vi "Handle Command.vi"(8 "error in (no error)":errorcluster, 9 "Data":variant, 10 "Command":string, 11 "Instrument.Lockin":refnum<class "Instrument.Lockin.lvclass">) -> (0 "error out":errorcluster, 1 "Processed Data":variant, 2 "Command":string, 3 "Instrument.Lockin out":refnum<class "Instrument.Lockin.lvclass">)   [LabVIEW 2019, in "Instrument.Lockin.lvlib" / "Instrument.Lockin.lvclass"]
uses:
  Instrument.Lockin.lvclass
  Typedefs/API/Lockin.Commands--Enum.ctl
  Typedefs/API/Lockin.Commands.Local--Enum.ctl
  <userlib>/LevyLab/Instrument Framework/Instrument Types/Lockin/Typedefs/LockinAPI.Sampling.Sampling--Cluster.ctl
  Instrument.Lockin.lvclass/Instrument.Lockin.ctl
  <userlib>/LevyLab/Instrument Framework/Instrument Types/Lockin/Typedefs/LockinAPI.Sampling.FsMode--enum.ctl
  <userlib>/LevyLab/Instrument Framework/Instrument Types/Lockin/Typedefs/LockinAPI.getState.states--enum.ctl
  <userlib>/LevyLab/Instrument Framework/Instrument Types/Lockin/Typedefs/LockinAPI.SweepData--Cluster.ctl
  Typedefs/API/Lockin.setState--cluster.ctl
  Instrument.DAQ/Typedefs/Set State-enum.ctl
  Typedefs/API/Lockin.setLogMode--cluster.ctl
  Typedefs/API/Lockin.setAO_Amp--cluster.ctl
  Typedefs/API/Lockin.setAO_DC--cluster.ctl
  Typedefs/API/Lockin.setAO_f--cluster.ctl
  Typedefs/API/Lockin.setAO_phi--cluster.ctl
  Typedefs/API/Lockin.setAO_function--cluster.ctl
  Instrument.DAQ/Typedefs/AO.Channel.Function--Enum.ctl
  Instrument.DAQ/Typedefs/AO.Channel--Cluster--Array.ctl
  Instrument.DAQ/Typedefs/AO.Channel--Cluster.ctl
  Typedefs/REF Parameter--Enum.ctl
  Typedefs/API/Lockin.setREF_f--cluster.ctl
  Typedefs/API/Lockin.setREF_phi--cluster.ctl
  Typedefs/API/Lockin.setREF_TC--cluster.ctl
  Typedefs/API/Lockin.setREF_RollOff--cluster.ctl
  Instrument.DAQ/Typedefs/REF.Channel--Cluster--Array.ctl
  Instrument.DAQ/Typedefs/REF.Channel--Cluster.ctl
  Instrument.DAQ/Typedefs/Sweep.Configuration--Cluster.ctl
  Instrument.DAQ/Typedefs/Sweep.Channel--Cluster--Array.ctl
  Instrument.DAQ/Typedefs/Sweep.Channel--Cluster.ctl
  Instrument.DAQ/Typedefs/Sweep.Pattern--Enum.ctl
  Typedefs/API/Lockin.setSweep_Time--cluster.ctl
  Typedefs/API/Lockin.setSweep_Table--cluster.ctl
  Instrument.DAQ/Typedefs/DAQ.Sampling.Sampling--Cluster.ctl
  Typedefs/API/Lockin.setSamplingFsMode--cluster.ctl
  Instrument.DAQ/Typedefs/DAQ.Sampling.Fs Mode--enum.ctl
  Instrument.DAQ/Typedefs/Channel.Gain--Cluster.ctl
  Instrument.DAQ/Typedefs/DAQ.Configuration--Cluster--Array.ctl
  Instrument.DAQ/Typedefs/DAQ.Configuration--Cluster.ctl
  Instrument.DAQ/Typedefs/DAQ.Config.AO.Range--enum.ctl
  Instrument.DAQ/Typedefs/DAQ.Config.AI.Range--enum.ctl
  Instrument.DAQ/Typedefs/DAQ.Config.AI.Coupling--enum.ctl
  Instrument.DAQ/Typedefs/PrivateEvents--DAQ.showUI.ctl
  Instrument.DAQ/Typedefs/AI.Channel--Cluster--Array.ctl
  Instrument.DAQ/Typedefs/AI.Channel--Cluster.ctl
  Instrument.DAQ/Typedefs/Simulation Mode--enum.ctl
  Typedefs/Offset Mode--Enum.ctl
  Instrument.DAQ/Typedefs/PrivateEvents--DAQ.setCalibration.ctl
  Instrument.DAQ/Typedefs/Configuration.Prefilter--Cluster.ctl
  Instrument.DAQ/Typedefs/Configuration.LinkFrequencies--Cluster.ctl
  Instrument.DAQ/Typedefs/Configuration.AmplitudeLimit--Cluster.ctl
  Typedefs/API/Lockin.setSamplingMode--cluster.ctl
  Instrument.DAQ/Typedefs/DAQ.Sampling.Sample Mode--Ring.ctl
  afc408c1-4a47-494c-817e-7b9f9bb33729.vi
  a7ccf487-04bf-437f-bc58-012293c091eb.vi
  06f5bff1-b823-416c-a758-fc672ecfcc99.vi
  029a7bc4-99e9-4f65-b437-c26585c9cd40.vi
  95117756-58c8-4cf5-b4a1-eea4f9571e2f.vi
  d527b0ad-2cbe-40d7-81d2-49d8d0078832.vi
  c6561379-f98d-4793-93aa-fc4f7b6fa2da.vi
  f7b28b50-f868-4d06-8d90-790d331e6843.vi
  3b890341-4124-4342-9d75-403cba162ea7.vi
  efd52b93-d691-4a9b-b54f-f4c6778ec2a4.vi
  1b48001d-6f4c-40ce-9883-2cfdfc5b0066.vi
  2465c698-e437-4a4f-8860-a626a4e5f6de.vi
  451a16e7-7f0f-4872-98b2-f896a68061ac.vi
  ce862ac6-3818-4682-989c-38fcf43d7c0a.vi
  0f1e83ab-c55c-46b9-bca3-9d617c6a026d.vi
  c46d61d8-ad78-4a4f-bd83-bba7d42c3393.vi
  06811b67-d74b-4972-af3b-9250fa170671.vi
  148daf87-aacf-4ea0-9f45-6b19ec731a12.vi
  b666889e-e9d3-40fa-bff7-b740bef29075.vi
  7fa0c9c7-d96f-42eb-b083-8fec20da1e25.vi
  2eef0b96-7480-46b2-a416-598848f5f946.vi
  4baefe16-dd55-4900-a34f-f85402a43af0.vi
  bf5afc16-6b2f-47bd-9035-54b404507785.vi
  df248ea2-cdbc-4a64-a66c-167358fcc18f.vi
  f4b2f717-a3e3-4701-aa1a-36f1ad587562.vi
  cb03029c-6dea-422e-9ff0-c01ba24202a7.vi
  ea7ae40a-427f-4df9-8330-54c2df2a5be0.vi
  d5077292-e533-4b52-a4d7-ebb5f6280e78.vi
  be7fa38f-04e0-4644-9c08-a6c1d8484273.vi
  228c5f99-5a8a-4ac9-8c3f-6c80f04cbb43.vi
  d91f965c-decf-4ad0-9779-3bd2f4599088.vi
  d9adaec0-ad08-4a9e-8669-6c491ae292cb.vi
  acd43294-18b9-4ae6-b527-f08772f90be2.vi
  6a1e6d83-5b10-4acb-978a-0f1ae3d31a35.vi
  847e6f07-fde4-45b3-9907-c341240c9864.vi
  b8b9aa39-8fbe-4465-abb6-4b3c602a596b.vi
  <vilib>/JDP Science/JSONtext/JSON text to Variant.vi
  <vilib>/JDP Science/JSONtext/LVClass Serializer/JSONtext LVClass Serializer.lvclass
  <userlib>/LevyLab/Instrument Framework/Instrument Types/Lockin/Instrument.LockinAPI.lvclass
  Instrument.DAQ/Instrument.DAQ.lvclass
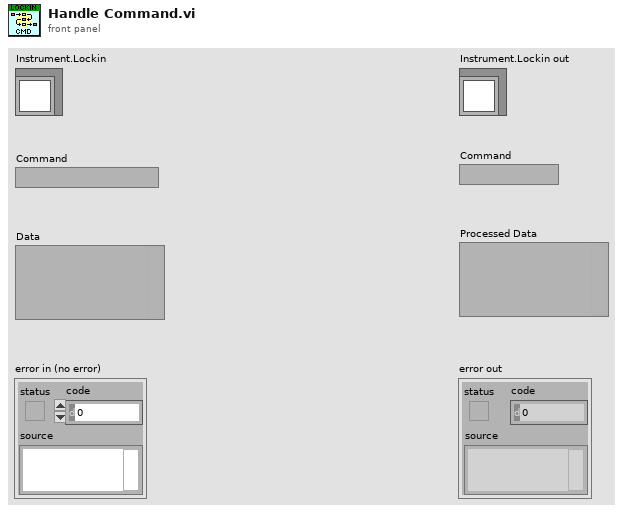
[diagram p1: front panel]
types:
  T1 = typedef "Instrument.Lockin.lvlib/Instrument.Lockin.lvclass/Lockin.Commands.Local--Enum.ctl" = enum16{"autoConfigureDAQ", "setSimulationMode", "zeroPhase", "setCalibration", "setPreFilter", "setLinkFrequencies", "setLimitAmplitude", "setLimitDC", "setSamplingDecimationPreDSP", "setSamplingDecimationPostDSP", "setSamplingMode", "setSamplingFsMultiplier", "setSamplingFsOutput", "setSamplingRefreshRate", "setData_State", "setData_DAQ", "setData_Sampling", "setData_Waveforms", "setData_Results", "setData_SweepWaveforms", "setData_AIChannels", "setData_AOChannels", "setData_REFChannels", "setData_InputGain", "setData_OutputGain", "showUI", "setAI", "setOffset", "setOffsetMode"}
  T2 = typedef "Instrument.Lockin.lvlib/Instrument.Lockin.lvclass/Lockin.Commands--Enum.ctl" = enum16{"setAO", "setAO_Amplitude", "setAO_DC", "setAO_Frequency", "setAO_Phase", "setAO_Function", "setREF", "setREF_Frequency", "setREF_Phase", "setREF_TC", "setREF_Roll-Off", "setDAQ", "setSampling", "setState", "getState", "getAO", "getAI", "getResults", "getSampling", "getAOconfig", "getREFconfig", "setInputGain", "setOutputGain", "getInputGain", "getOutputGain", "setSamplingFsMode", "getSamplingFsMode", "setSweep", "setSweep_Time", "setSweep_Table", "getStatus", "getSweepResults", "getSweepWaveforms", "startLogging", "stopLogging"}
  T3 = typedef "Instrument.LockinAPI.lvclass/LockinAPI.Sampling.Sampling--Cluster.ctl" = cluster{"Fs":dbl, "#s":i32}
  T4 = typedef "Instrument.LockinAPI.lvclass/LockinAPI.getState.states--enum.ctl" = enum16{"idle", "created", "started", "stopped", "sweeping"}
  T5 = typedef "Instrument.LockinAPI.lvclass/LockinAPI.SweepData--Cluster.ctl" = cluster{"AO":waveform(dbl)[], "AI":waveform(dbl)[], "X":waveform(dbl)[], "Y":waveform(dbl)[]}
  T6 = typedef "Instrument.Lockin.lvlib/Instrument.Lockin.lvclass/Lockin.setState--cluster.ctl" = cluster{"State":T7}
  T7 = typedef "Instrument.Lockin.lvlib/Instrument.DAQ.lvclass/Set State-enum.ctl" = enum16{"start", "stop", "reset", "start sweep", "stop sweep"}
  T8 = typedef "Instrument.Lockin.lvlib/Instrument.Lockin.lvclass/Lockin.setLogMode--cluster.ctl" = cluster{"interval":u32}
  T9 = enum16{"Amplitude", "DC", "Frequency", "Phase", "Function"}
  T10 = typedef "Instrument.Lockin.lvlib/Instrument.Lockin.lvclass/Lockin.setAO_Amp--cluster.ctl" = cluster{"Channel":i32, "Amplitude":dbl}
  T11 = typedef "Instrument.Lockin.lvlib/Instrument.Lockin.lvclass/Lockin.setAO_DC--cluster.ctl" = cluster{"Channel":i32, "DC":dbl}
  T12 = typedef "Instrument.Lockin.lvlib/Instrument.Lockin.lvclass/Lockin.setAO_f--cluster.ctl" = cluster{"Channel":i32, "Frequency":dbl}
  T13 = typedef "Instrument.Lockin.lvlib/Instrument.Lockin.lvclass/Lockin.setAO_phi--cluster.ctl" = cluster{"Channel":i32, "Phase":dbl}
  T14 = typedef "Instrument.Lockin.lvlib/Instrument.Lockin.lvclass/Lockin.setAO_function--cluster.ctl" = cluster{"Channel":i32, "Function":T15}
  T15 = typedef "Instrument.Lockin.lvlib/Instrument.DAQ.lvclass/AO.Channel.Function--Enum.ctl" = enum16{"Sine", "Triangle", "Square"}
  T16 = typedef "Instrument.Lockin.lvlib/Instrument.DAQ.lvclass/AO.Channel--Cluster--Array.ctl" = T17[]
  T17 = typedef "Instrument.Lockin.lvlib/Instrument.DAQ.lvclass/AO.Channel--Cluster.ctl" = cluster{"Enable?":bool, "Channel":i32, "Amplitude":dbl, "Offset":dbl, "Frequency":dbl, "Phase":dbl, "Function":T15, "Sweeping?":bool}
  T18 = typedef "Instrument.Lockin.lvlib/Instrument.Lockin.lvclass/Lockin.setREF_f--cluster.ctl" = cluster{"Channel":i32, "Frequency":dbl}
  T19 = typedef "Instrument.Lockin.lvlib/Instrument.Lockin.lvclass/REF Parameter--Enum.ctl" = enum16{"Frequency", "Phase", "Time Constant", "RollOff"}
  T20 = typedef "Instrument.Lockin.lvlib/Instrument.Lockin.lvclass/Lockin.setREF_phi--cluster.ctl" = cluster{"Channel":i32, "Phase":dbl}
  T21 = typedef "Instrument.Lockin.lvlib/Instrument.Lockin.lvclass/Lockin.setREF_TC--cluster.ctl" = cluster{"Channel":i32, "TC":dbl}
  T22 = typedef "Instrument.Lockin.lvlib/Instrument.Lockin.lvclass/Lockin.setREF_RollOff--cluster.ctl" = cluster{"Channel":i32, "Roll-Off":i32}
  T23 = typedef "Instrument.Lockin.lvlib/Instrument.DAQ.lvclass/REF.Channel--Cluster--Array.ctl" = T24[]
  T24 = typedef "Instrument.Lockin.lvlib/Instrument.DAQ.lvclass/REF.Channel--Cluster.ctl" = cluster{"Enable?":bool, "Channel":i32, "Frequency":dbl, "Phase":dbl, "TC":dbl, "Roll-Off":i32}
  T25 = typedef "Instrument.Lockin.lvlib/Instrument.Lockin.lvclass/Lockin.setSweep_Time--cluster.ctl" = cluster{"SweepTime":dbl}
  T26 = typedef "Instrument.Lockin.lvlib/Instrument.Lockin.lvclass/Lockin.setSweep_Table--cluster.ctl" = cluster{"Channel":i32, "Table":dbl[]}
  T27 = typedef "Instrument.Lockin.lvlib/Instrument.DAQ.lvclass/DAQ.Sampling.Sampling--Cluster.ctl" = cluster{"Fs":dbl, "#s":i32}
  T28 = typedef "Instrument.Lockin.lvlib/Instrument.Lockin.lvclass/Lockin.setSamplingFsMode--cluster.ctl" = cluster{"FsMode":T29}
  T29 = typedef "Instrument.Lockin.lvlib/Instrument.DAQ.lvclass/DAQ.Sampling.Fs Mode--enum.ctl" = enum16{"Manual", "Auto Fs", "Max Fs"}
  T30 = typedef "Instrument.Lockin.lvlib/Instrument.DAQ.lvclass/Channel.Gain--Cluster.ctl" = cluster{"Channel":string, "Gain":dbl}
  T31 = typedef "Instrument.Lockin.lvlib/Instrument.DAQ.lvclass/DAQ.Configuration--Cluster--Array.ctl" = T32[]
  T32 = typedef "Instrument.Lockin.lvlib/Instrument.DAQ.lvclass/DAQ.Configuration--Cluster.ctl" = cluster{"Device":string, "AO.Ch":string, "AO.Range":T33, "AI.Ch":string, "AI.Range":T34, "AI.Coupling":T35}
  T33 = typedef "Instrument.Lockin.lvlib/Instrument.DAQ.lvclass/DAQ.Config.AO.Range--enum.ctl" = enum16{"±0.1", "±1.0", "±10.0"}
  T34 = typedef "Instrument.Lockin.lvlib/Instrument.DAQ.lvclass/DAQ.Config.AI.Range--enum.ctl" = enum16{"±0.316", "±1.00", "±3.16", "±10.0", "±31.6", "±42.4"}
  T35 = typedef "Instrument.Lockin.lvlib/Instrument.DAQ.lvclass/DAQ.Config.AI.Coupling--enum.ctl" = u16
  T36 = typedef "Instrument.Lockin.lvlib/Instrument.DAQ.lvclass/PrivateEvents--DAQ.showUI.ctl" = bool
  T37 = typedef "Instrument.Lockin.lvlib/Instrument.DAQ.lvclass/AI.Channel--Cluster--Array.ctl" = T38[]
  T38 = typedef "Instrument.Lockin.lvlib/Instrument.DAQ.lvclass/AI.Channel--Cluster.ctl" = cluster{"Enable?":bool, "Channel":i32, "References":i32[]}
  T39 = typedef "Instrument.Lockin.lvlib/Instrument.DAQ.lvclass/Simulation Mode--enum.ctl" = enum16{"AI = HW simulated", "AI = noise*AO", "AI = waveguide"}
  T40 = typedef "Instrument.Lockin.lvlib/Instrument.Lockin.lvclass/Offset Mode--Enum.ctl" = enum16{"Measure", "Remove"}
  T41 = typedef "Instrument.Lockin.lvlib/Instrument.DAQ.lvclass/PrivateEvents--DAQ.setCalibration.ctl" = enum16{"Check", "Calibrate"}
  T42 = typedef "Instrument.Lockin.lvlib/Instrument.DAQ.lvclass/Configuration.Prefilter--Cluster.ctl" = cluster{"60 Hz":bool, "Low Pass":bool, "Low Pass Cutoff (Hz)":dbl}
  T43 = typedef "Instrument.Lockin.lvlib/Instrument.DAQ.lvclass/Configuration.LinkFrequencies--Cluster.ctl" = cluster{"Link?":bool, "Frequency (Hz)":dbl}
  T44 = typedef "Instrument.Lockin.lvlib/Instrument.Lockin.lvclass/Lockin.setSamplingMode--cluster.ctl" = cluster{"SampleMode":T45}
  T45 = typedef "Instrument.Lockin.lvlib/Instrument.DAQ.lvclass/DAQ.Sampling.Sample Mode--Ring.ctl" = i32
  T46 = typedef "Instrument.LockinAPI.lvclass/LockinAPI.Sampling.FsMode--enum.ctl" = enum16{"Manual", "Auto Fs", "Max Fs"}
  T47 = typedef "Instrument.Lockin.lvlib/Instrument.DAQ.lvclass/Get State-enum.ctl" = enum16{"idle", "created", "started", "stopped", "sweeping"}
  T48 = typedef "Instrument.Lockin.lvlib/Instrument.DAQ.lvclass/Channel.Gain--Cluster--Array.ctl" = T30[]
  T49 = typedef "Instrument.Lockin.lvlib/Instrument.DAQ.lvclass/Results--Cluster.ctl" = cluster{"Time Stamp":timestamp, "Results (Dictionary)":cluster{"key":string, "value":dbl}[]}
  T50 = typedef "Instrument.Lockin.lvlib/Instrument.DAQ.lvclass/Sweep.Configuration--Cluster.ctl" = cluster{"Sweep Time (s)":dbl, "Initial Wait (s)":dbl, "Return to Start":bool, "Channels":T51}
  T51 = typedef "Instrument.Lockin.lvlib/Instrument.DAQ.lvclass/Sweep.Channel--Cluster--Array.ctl" = T52[]
  T52 = typedef "Instrument.Lockin.lvlib/Instrument.DAQ.lvclass/Sweep.Channel--Cluster.ctl" = cluster{"Enable?":bool, "Channel":u16, "Start":dbl, "End":dbl, "Pattern":T53, "Table":dbl[]}
  T53 = typedef "Instrument.Lockin.lvlib/Instrument.DAQ.lvclass/Sweep.Pattern--Enum.ctl" = enum16{"Ramp /", "Ramp /\\", "Smooth Ramp _/", "Smooth Ramp _/\\_", "Table"}
  T54 = typedef "Instrument.Lockin.lvlib/Instrument.DAQ.lvclass/DAQ.Sampling--Cluster.ctl" = cluster{"Sampling":T27, "sample mode":i32, "Fs Mode":T29, "Fs Multiplier":dbl, "Refresh Rate (Hz)":dbl, "Decimation.PreDSP":i32, "Decimation.PostDSP":i32, "Fs.Output":dbl}
  T55 = typedef "Instrument.Lockin.lvlib/Instrument.DAQ.lvclass/DAQ.Config.AO--Cluster--Array.ctl" = T56[]
  T56 = typedef "Instrument.Lockin.lvlib/Instrument.DAQ.lvclass/DAQ.Config.AO--Cluster.ctl" = cluster{"Channels":tag, "Range":T33, "output terminal configuration":i32, "Type":T57}
  T57 = typedef "Instrument.Lockin.lvlib/Instrument.DAQ.lvclass/DAQ.Type--enum.ctl" = enum16{"None", "USB-4431", "PXI-446x"}
  T58 = typedef "Instrument.Lockin.lvlib/Instrument.DAQ.lvclass/DAQ.Config.AI--Cluster--Array.ctl" = T59[]
  T59 = typedef "Instrument.Lockin.lvlib/Instrument.DAQ.lvclass/DAQ.Config.AI--Cluster.ctl" = cluster{"Channels":tag, "Coupling":T35, "Range":T34, "input terminal configuration":i32, "Type":T57}
  T60 = typedef "Instrument.Lockin.lvlib/Instrument.DAQ.lvclass/PublicEvents--DAQ.getWaveforms.ctl" = cluster{"AO_wfm":waveform(dbl)[], "AI_wfm":waveform(dbl)[], "Ref_X_wfm":waveform(dbl)[], "Ref_Y_wfm":waveform(dbl)[], "X_wfm":waveform(dbl)[], "Y_wfm":waveform(dbl)[]}
  T61 = typedef "Instrument.Lockin.lvlib/Instrument.DAQ.lvclass/PublicEvents--DAQ.getSweepWaveforms.ctl" = cluster{"AO_wfm":waveform(dbl)[], "AI_wfm":waveform(dbl)[], "X_wfm":waveform(dbl)[], "Y_wfm":waveform(dbl)[]}
  T62 = typedef "Instrument.Lockin.lvlib/Instrument.DAQ.lvclass/Configuration.AmplitudeLimit--Cluster.ctl" = cluster{"Limit?":bool, "Limit (V)":dbl}
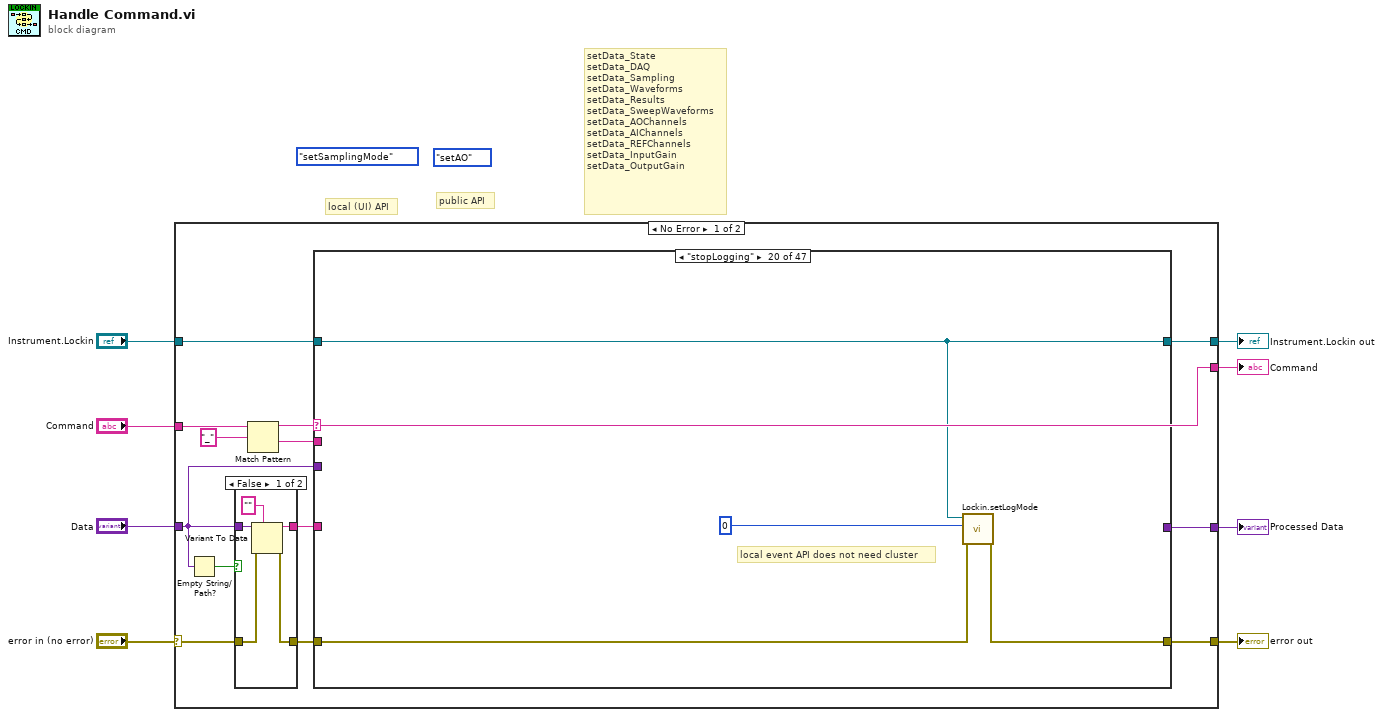
[diagram p0: block diagram]
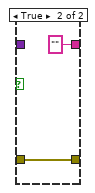
[diagram p2: hidden frame]
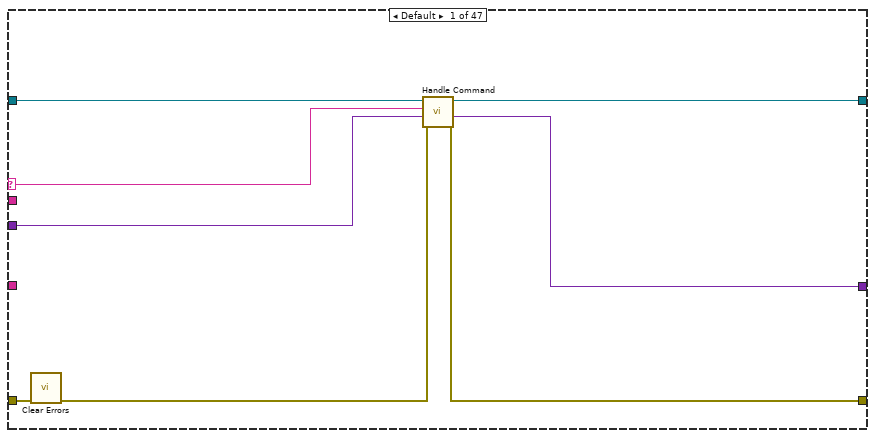
[diagram p3: hidden frame]
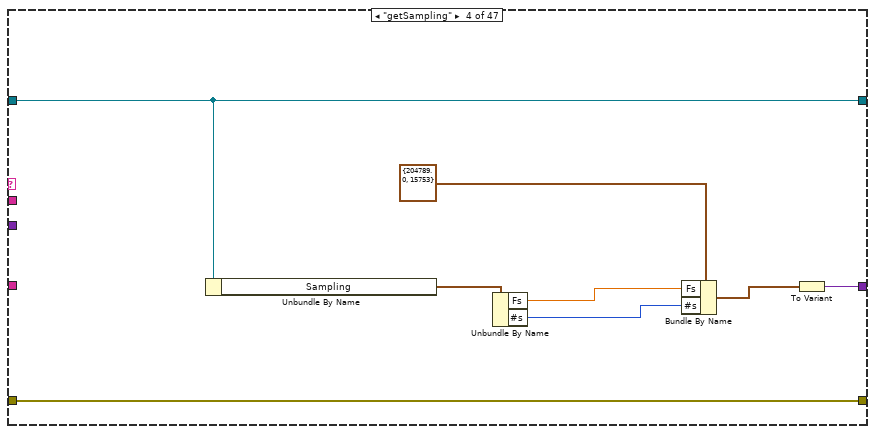
[diagram p6: hidden frame]
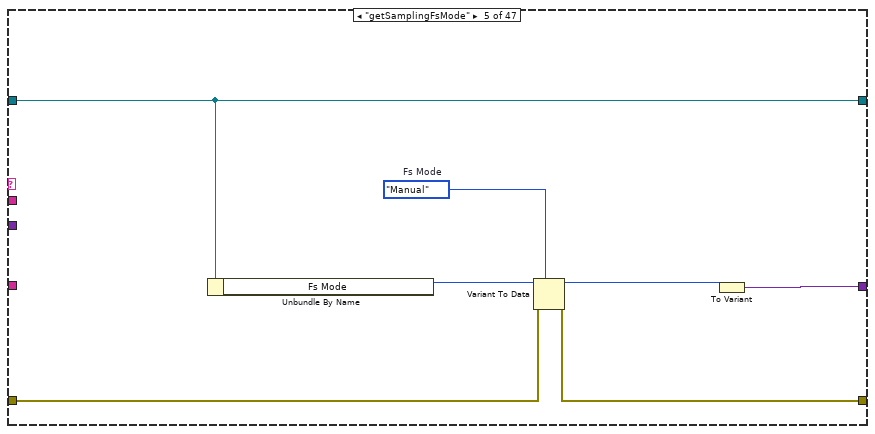
[diagram p7: hidden frame]
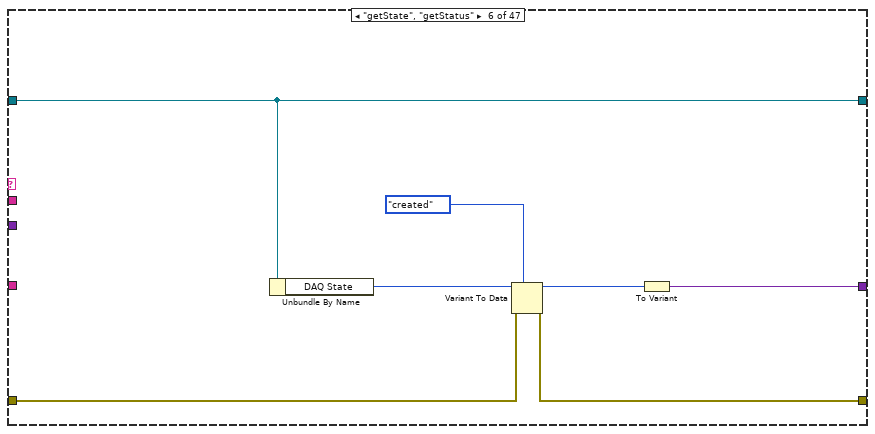
[diagram p8: hidden frame]
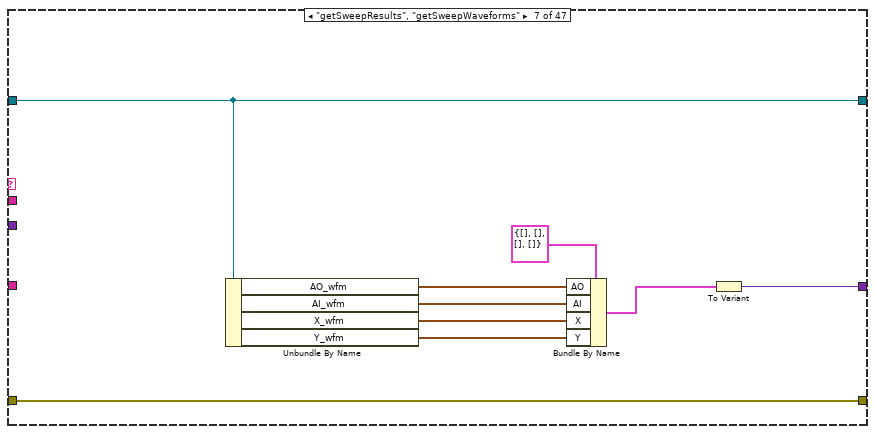
[diagram p9: hidden frame]
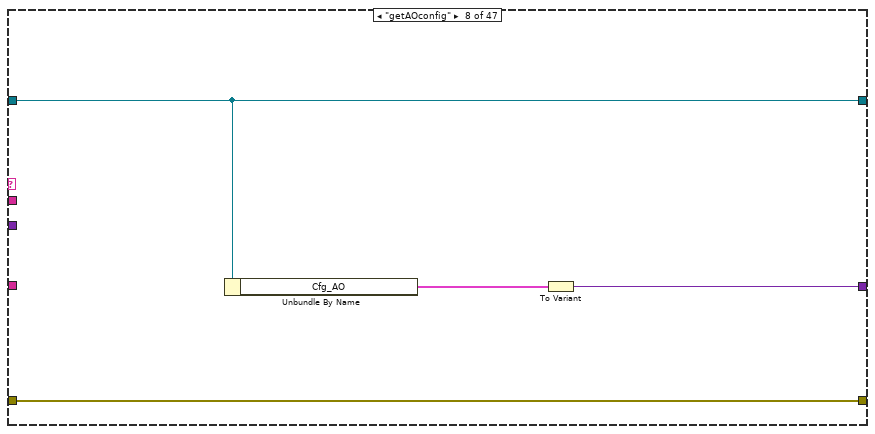
[diagram p10: hidden frame]
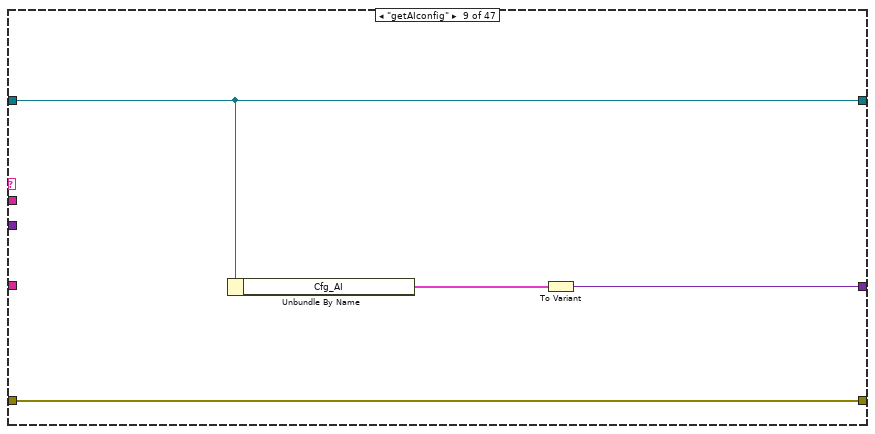
[diagram p11: hidden frame]
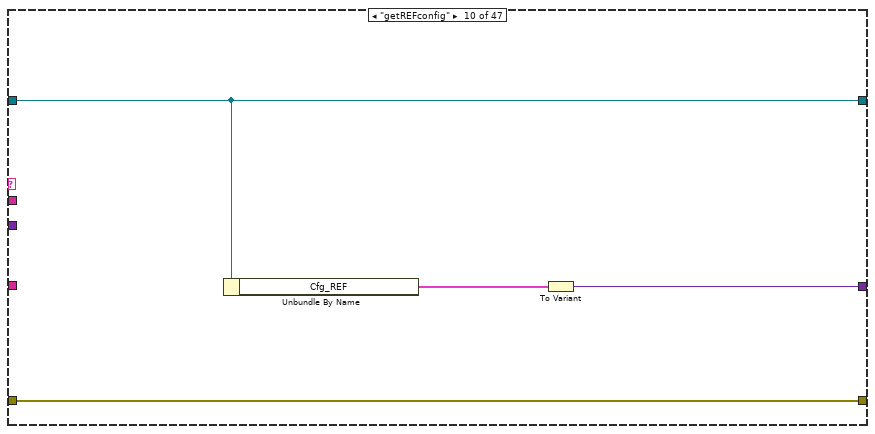
[diagram p12: hidden frame]
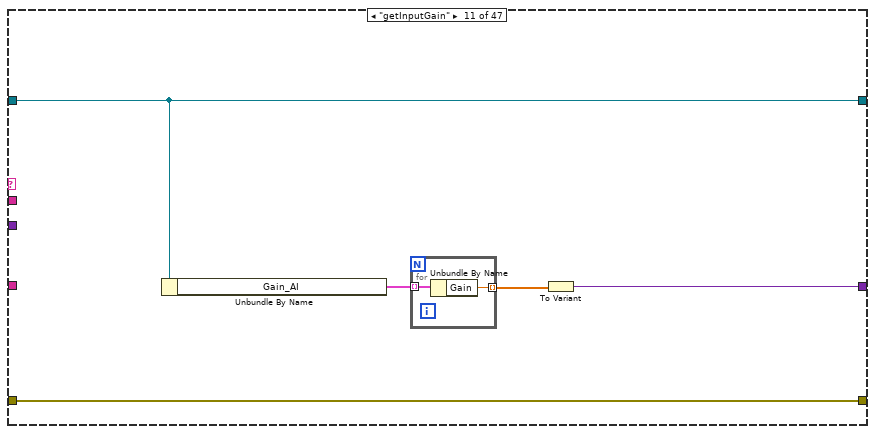
[diagram p13: hidden frame]
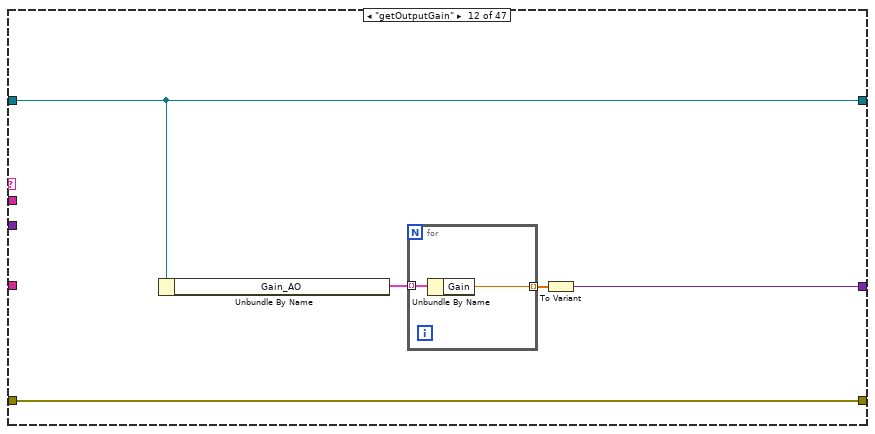
[diagram p14: hidden frame]
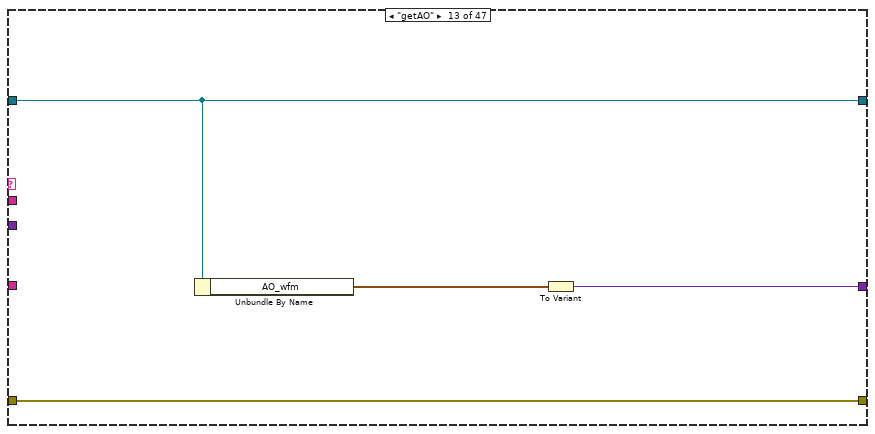
[diagram p15: hidden frame]
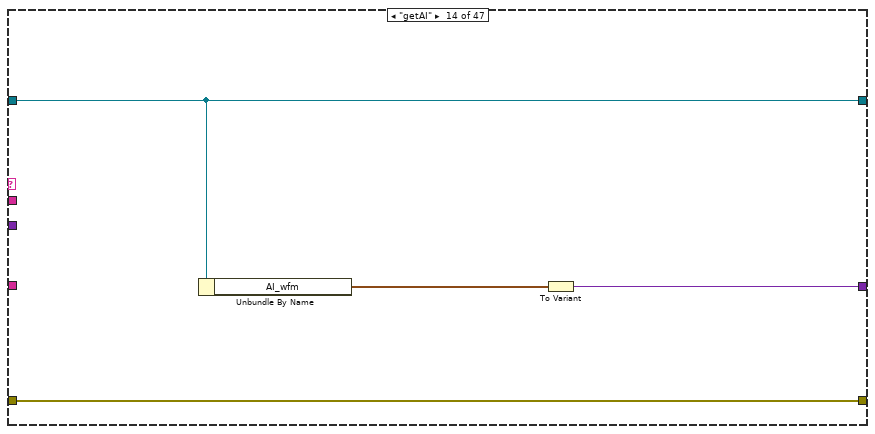
[diagram p16: hidden frame]
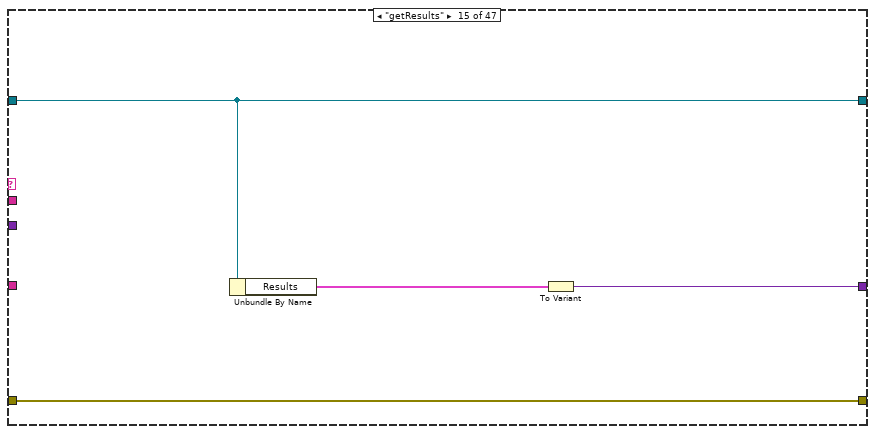
[diagram p17: hidden frame]
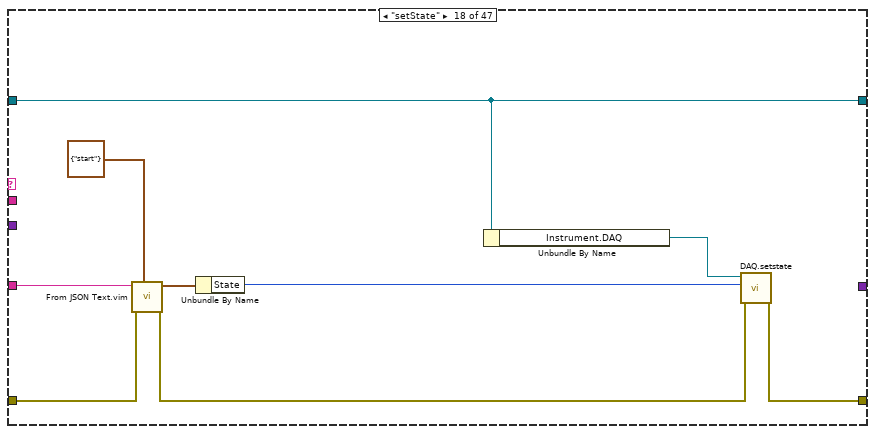
[diagram p20: hidden frame]
diagram:
  (unwired) Lockin.Commands.Local--Enum."setSamplingMode" ("Enum")
  (unwired) Lockin.Commands--Enum."setAO" ("Enum")
  # "setData_State\nsetData_DAQ\nsetData_Sampling\nsetData_Waveforms\nsetData_Results\nsetData_SweepWaveforms\nsetData_AOChannels\nsetData_AIChannels\nsetData_REFChannels\nsetData_InputGain\nsetData_OutputGain"
  # "local (UI) API"
  # "public API"
  n1 = case shown="No Error" "error in (no error)" {
    selector: "error in (no error)" -> [w17 w662]
    tunnel: [w18 w662] -> w7
    tunnel: [w20 w661] -> w6
    tunnel: "Instrument.Lockin" -> [w21 w661]
    tunnel: "Command" -> [w12 w660]
    tunnel: [w19 variant] -> w5
    tunnel: "Data" -> [w9 _]
    tunnel: [w11 w660] -> w3
    frame No Error {
      n2 = Empty String/Path?(string/path=w9) -> (empty?=w10:bool)
      n3 = case shown="False" w10 {
        tunnel: w17 -> [w26 w27]
        tunnel: [w24 ""] -> w16
        tunnel: [w23 w27] -> w13
        tunnel: w9 -> [w22 _]
        frame False {
          n4 = Variant To Data(error in=w26, type="", Variant=w22) -> (data=w24:string, error out=w23:errorcluster)
        }
        frame True {
        }
      }
      n5 = Match Pattern(string=w12, regular expression="_") -> (before substring=w11:string, after substring=w14:string)  [unwired: 1 in, 2 out]
      n6 = case shown="\"stopLogging\"" w11 {
        selector: w11 -> [w31 _ _ _ _ _ _ _ _ _ _ _ _ _ _ _ _ _ _ _ _ _ _ _ _ _ _ _ _ _ _ _ _ _ _ _ _ _ _ _ _ _ _ _ _ _ _]
        tunnel: w21 -> [w36 w38 w40 w46 w54 w61 w69 w72 w76 w80 w86 w93 w98 w102 w106 w111 w113 w117 w126 w134 w139 w213 w272 w304 w319 w328 w346 w365 w382 w395 w397 w411 w419 w526 w539 w549 w558 w567 w574 w586 w596 w604 w614 w628 w638 w648 w658]
        tunnel: [w34 w38 w40 w46 w54 w61 w69 w72 w76 w80 w86 w93 w98 w102 w106 w111 w113 w117 w126 w134 w137 w208 w276 w303 w316 w329 w347 w366 w381 w395 w397 w405 w415 w526 w538 w549 w558 w567 w575 w587 w597 w603 w613 w625 w635 w645 w655] -> w20
        tunnel: [w35 _ _ w48 w55 w62 w71 w74 w78 w82 w88 w95 w101 w105 w109 _ _ _ _ _ _ _ _ _ _ _ _ _ _ _ _ _ _ _ _ w540 _ _ _ _ _ _ _ _ _ _ _] -> w19
        tunnel: w16 -> [_ _ _ _ _ _ _ _ _ _ _ _ _ _ _ _ _ w122 w130 _ w143 w216 w280 w310 w321 w334 w352 w370 w393 _ w403 w413 w417 _ w533 w546 _ w564 w571 w582 w592 w602 w612 w623 w632 w642 w653]
        tunnel: [w32 w37 w39 w47 w50 w57 w70 w73 w77 w81 w87 w94 w100 w104 w108 w110 w112 w118 w123 w133 w140 w209 w277 w306 w314 w330 w348 w367 w387 w394 w398 w407 w414 w528 w534 w547 w556 w565 w576 w583 w593 w605 w615 w624 w634 w644 w654] -> w18
        tunnel: w14 -> [_ _ _ _ _ _ _ _ _ _ _ _ _ _ _ _ _ _ _ _ w138 w214 w273 _ _ _ _ _ _ _ _ _ w418 _ _ _ _ _ _ _ _ _ _ _ _ _ _]
        tunnel: w13 -> [w33 w37 w39 w47 w49 w56 w70 w73 w77 w81 w87 w94 w100 w104 w108 w110 w112 w121 w129 w131 w142 w215 w279 w308 w320 w333 w351 w369 w392 w394 w400 w412 w416 w527 w532 w543 w557 w560 w569 w580 w589 w601 w611 w622 w630 w641 w650]
        tunnel: w9 -> [w30 _ _ _ _ _ _ _ _ _ _ _ _ _ _ _ _ _ _ _ _ _ _ _ _ _ _ _ _ _ _ _ _ _ _ _ _ _ _ _ _ _ _ _ _ _ _]
        frame Default {
          n7 = call <vilib>:"Clear Errors.vi"("error in (no error)"=w33) -> ("error out"=w29:errorcluster)  [unwired: 5 in, 1 out]
          n8 = call-parent "Handle Command.vi"("error in (no error)"=w29, "params in"=w30, "command"=w31, "Instrument in"=w36) -> ("error out"=w32:errorcluster, "processed data"=w35:variant, "Instrument out"=w34:refnum<class "Instrument.Lockin.lvclass">)  [unwired: 4 in, 1 out]
        }
        frame "----------PUBLIC API----------" {
        }
        frame "----------GET METHODS----------" {
        }
        frame "getSampling" {
          n9 = Unbundle By Name(w46) -> ("Sampling"=w44:T27)
          n10 = Unbundle By Name(w44) -> ("Fs"=w43:dbl, "#s"=w42:i32)
          n11 = Bundle By Name(cluster=T3 {"Fs"=204789.0, "#s"=15753} ("sampling"), "Fs"=w43, "#s"=w42) -> (w41:T3)
          n12 = To Variant(anything=w41) -> (Variant=w48:variant)
        }
        frame "getSamplingFsMode" {
          w52 = LockinAPI.Sampling.FsMode--enum."Manual"  # Fs Mode
          n13 = Unbundle By Name(w54) -> ("Fs Mode"=w53:T29)
          n14 = Variant To Data(error in=w49, type=w52, Variant=w53) -> (data=w51:T46, error out=w50:errorcluster)
          n15 = To Variant(anything=w51) -> (Variant=w55:variant)
        }
        frame "getState", "getStatus" {
          n16 = Unbundle By Name(w61) -> ("DAQ State"=w59:T47)
          n17 = Variant To Data(error in=w56, type=LockinAPI.getState.states--enum."created" ("getState.states"), Variant=w59) -> (data=w58:T4, error out=w57:errorcluster)
          n18 = To Variant(anything=w58) -> (Variant=w62:variant)
        }
        frame "getSweepResults", "getSweepWaveforms" {
          n19 = Unbundle By Name(w69) -> ("AO_wfm"=w67:waveform(dbl)[], "AI_wfm"=w66:waveform(dbl)[], "X_wfm"=w65:waveform(dbl)[], "Y_wfm"=w64:waveform(dbl)[])
          n20 = Bundle By Name(cluster=T5 {"AO"=[], "AI"=[], "X"=[], "Y"=[]} ("sweepData"), "AO"=w67, "AI"=w66, "X"=w65, "Y"=w64) -> (w63:T5)
          n21 = To Variant(anything=w63) -> (Variant=w71:variant)
        }
        frame "getAOconfig" {
          n22 = Unbundle By Name(w72) -> ("Cfg_AO"=w75:T16)
          n23 = To Variant(anything=w75) -> (Variant=w74:variant)
        }
        frame "getAIconfig" {
          n24 = Unbundle By Name(w76) -> ("Cfg_AI"=w79:T37)
          n25 = To Variant(anything=w79) -> (Variant=w78:variant)
        }
        frame "getREFconfig" {
          n26 = Unbundle By Name(w80) -> ("Cfg_REF"=w83:T23)
          n27 = To Variant(anything=w83) -> (Variant=w82:variant)
        }
        frame "getInputGain" {
          n28 = Unbundle By Name(w86) -> ("Gain_AI"=w85:T48)
          n29 = for {
            tunnel: w85 -> [w90] mode=indexing
            tunnel: [w89] -> w84 mode=indexing
            n30 = Unbundle By Name(w90) -> ("Gain"=w89:dbl)
          }
          n31 = To Variant(anything=w84) -> (Variant=w88:variant)
        }
        frame "getOutputGain" {
          n32 = Unbundle By Name(w93) -> ("Gain_AO"=w92:T48)
          n33 = for {
            tunnel: w92 -> [w97] mode=indexing
            tunnel: [w96] -> w91 mode=indexing
            n34 = Unbundle By Name(w97) -> ("Gain"=w96:dbl)
          }
          n35 = To Variant(anything=w91) -> (Variant=w95:variant)
        }
        frame "getAO" {
          n36 = Unbundle By Name(w98) -> ("AO_wfm"=w99:waveform(dbl)[])
          n37 = To Variant(anything=w99) -> (Variant=w101:variant)
        }
        frame "getAI" {
          n38 = Unbundle By Name(w102) -> ("AI_wfm"=w103:waveform(dbl)[])
          n39 = To Variant(anything=w103) -> (Variant=w105:variant)
        }
        frame "getResults" {
          n40 = Unbundle By Name(w106) -> ("Results"=w107:T49)
          n41 = To Variant(anything=w107) -> (Variant=w109:variant)
        }
        frame "getAUX" {
        }
        frame "----------SET METHODS----------" {
        }
        frame "setState" {
          n42 = call "From JSON Text.vim"("Data Type and Default Value"=T6 {"State"=enum."start"} ("setState"), "error in (no error)"=w121, "JSON"=w122) -> ("error out"=w119:errorcluster, "Data out"=w115:T6)  [unwired: 7 in]
          n43 = Unbundle By Name(w115) -> ("State"=w114:T7)
          n44 = Unbundle By Name(w117) -> ("Instrument.DAQ"=w120:refnum<class "Instrument.DAQ.lvclass">)
          n45 = call "DAQ.setstate.vi"("error in (no error)"=w119, "setState"=w114, "Instrument.DAQ"=w120) -> ("error out"=w118:errorcluster)  [unwired: 7 in, 1 out]
        }
        frame "startLogging" {
          # "local event API does not need cluster"
          # "remote API store data in cluster"
          n46 = call "From JSON Text.vim"("Data Type and Default Value"=T8 {"interval"=1} ("setLogMode"), "error in (no error)"=w129, "JSON"=w130) -> ("error out"=w124:errorcluster, "Data out"=w128:T8)  [unwired: 7 in]
          n47 = Unbundle By Name(w128) -> ("interval"=w125:u32)
          n48 = call "Lockin.setLogMode.vi"("error in (no error)"=w124, "interval (ms)"=w125, "Instrument.Lockin"=w126) -> ("error out"=w123:errorcluster)  [unwired: 7 in, 1 out]
        }
        frame "stopLogging" {
          # "local event API does not need cluster"
          n49 = call "Lockin.setLogMode.vi"("error in (no error)"=w131, "interval (ms)"=u32 0 ("interval"), "Instrument.Lockin"=w134) -> ("error out"=w133:errorcluster)  [unwired: 7 in, 1 out]
        }
        frame "setAO" {
          # "Lockin SMO: Set AO"
          # "Adjust Channels"
          n50 = case shown="\"\"" w138 {
            selector: w138 -> [w153 _]
            tunnel: w143 -> [w152 w205]
            tunnel: w142 -> [w151 w204]
            tunnel: [w146 w200] -> w136
            tunnel: w139 -> [w149 w203]
            tunnel: [w150 w202] -> w137
            frame Default {
              n51 = case shown="\"Phase\"" w153 {
                tunnel: w152 -> [w162 w171 w180 w189 w198]
                tunnel: w151 -> [w161 w170 w179 w188 w197]
                tunnel: [w160 w169 w178 w187 w196] -> w147
                tunnel: [T9."Amplitude" ("Parameter") T9."DC" ("Parameter") T9."Frequency" ("Parameter") T9."Phase" ("Parameter") T9."Function" ("Parameter")] -> w148
                tunnel: [w156 w166 w175 w184 w193] -> w145
                tunnel: [w154 w163 w172 w181 w190] -> w144
                frame "Amplitude", Default {
                  n52 = call "From JSON Text.vim"("Data Type and Default Value"=T10 {"Channel"=5, "Amplitude"=0.0} ("setAO_Amp"), "error in (no error)"=w161, "JSON"=w162) -> ("error out"=w160:errorcluster, "Data out"=w158:T10)  [unwired: 7 in]
                  n53 = Unbundle By Name(w158) -> ("Channel"=w156:i32, "Amplitude"=w155:dbl)
                  n54 = To Variant(anything=w155) -> (Variant=w154:variant)
                }
                frame "DC" {
                  n55 = call "From JSON Text.vim"("Data Type and Default Value"=T11 {"Channel"=5, "DC"=0.0} ("setAO_DC"), "error in (no error)"=w170, "JSON"=w171) -> ("error out"=w169:errorcluster, "Data out"=w168:T11)  [unwired: 7 in]
                  n56 = Unbundle By Name(w168) -> ("Channel"=w166:i32, "DC"=w165:dbl)
                  n57 = To Variant(anything=w165) -> (Variant=w163:variant)
                }
                frame "Frequency" {
                  n58 = call "From JSON Text.vim"("Data Type and Default Value"=T12 {"Channel"=5, "Frequency"=0.0} ("setAO_f"), "error in (no error)"=w179, "JSON"=w180) -> ("error out"=w178:errorcluster, "Data out"=w177:T12)  [unwired: 7 in]
                  n59 = Unbundle By Name(w177) -> ("Channel"=w175:i32, "Frequency"=w174:dbl)
                  n60 = To Variant(anything=w174) -> (Variant=w172:variant)
                }
                frame "Phase" {
                  n61 = call "From JSON Text.vim"("Data Type and Default Value"=T13 {"Channel"=5, "Phase"=0.0} ("setAO_phi"), "error in (no error)"=w188, "JSON"=w189) -> ("error out"=w187:errorcluster, "Data out"=w186:T13)  [unwired: 7 in]
                  n62 = Unbundle By Name(w186) -> ("Channel"=w184:i32, "Phase"=w183:dbl)
                  n63 = To Variant(anything=w183) -> (Variant=w181:variant)
                }
                frame "Function" {
                  n64 = call "From JSON Text.vim"("Data Type and Default Value"=T14 {"Channel"=5, "Function"=enum."Sine"} ("setAO_function"), "error in (no error)"=w197, "JSON"=w198) -> ("error out"=w196:errorcluster, "Data out"=w195:T14)  [unwired: 7 in]
                  n65 = Unbundle By Name(w195) -> ("Channel"=w193:i32, "Function"=w192:T15)
                  n66 = To Variant(anything=w192) -> (Variant=w190:variant)
                }
              }
              n67 = call "Update AO Parameter.vi"("Parameter"=w148, "error in"=w147, "Value"=w144, "Channel"=w145, "Instrument.Lockin"=w149) -> ("error out"=w146:errorcluster, "Instrument.Lockin out"=w150:refnum<class "Instrument.Lockin.lvclass">)  [unwired: 5 in]
            }
            frame "" {
              n68 = call "From JSON Text.vim"("Data Type and Default Value"=T16 [] ("AO Channels"), "error in (no error)"=w204, "JSON"=w205) -> ("error out"=w200:errorcluster, "Data out"=w201:T16)  [unwired: 7 in]
              n69 = Bundle By Name(cluster=w203, "Cfg_AO"=w201) -> (w202:refnum<class "Instrument.Lockin.lvclass">)
            }
          }
          n70 = Unbundle By Name(w137) -> ("Instrument.DAQ"=w141:refnum<class "Instrument.DAQ.lvclass">, "Cfg_AO"=w135:T16)
          n71 = call "DAQ.setAO.vi"("error in (no error)"=w136, "AO Channels"=w135, "Instrument.DAQ"=w141) -> ("error out"=w140:errorcluster)  [unwired: 7 in, 1 out]
        }
        frame "setREF" {
          # "Lockin SMO: Reset Phase"
          # "Lockin SMO: Set REF"
          # "Adjust Channels"
          n72 = case shown="Default" w214 {
            selector: w214 -> [w226 _]
            tunnel: w216 -> [w225 w269]
            tunnel: w215 -> [w224 w268]
            tunnel: [w221 w264] -> w207
            tunnel: w213 -> [w223 w267]
            tunnel: [w222 w266] -> w208
            frame Default {
              n73 = case shown="\"Frequency\", Default" w226 {
                tunnel: w225 -> [w235 w244 w253 w262]
                tunnel: w224 -> [w234 w243 w252 w261]
                tunnel: [w233 w242 w251 w260] -> w219
                tunnel: [REF_Parameter--Enum."Frequency" ("Parameter") REF_Parameter--Enum."Phase" ("Parameter") REF_Parameter--Enum."Time Constant" ("Parameter") REF_Parameter--Enum."RollOff" ("Parameter")] -> w220
                tunnel: [w231 w240 w249 w258] -> w217
                tunnel: [w229 w238 w247 w256] -> w218
                frame "Frequency", Default {
                  n74 = call "From JSON Text.vim"("Data Type and Default Value"=T18 {"Channel"=0, "Frequency"=0.0} ("setREF_f"), "error in (no error)"=w234, "JSON"=w235) -> ("error out"=w233:errorcluster, "Data out"=w232:T18)  [unwired: 7 in]
                  n75 = Unbundle By Name(w232) -> ("Channel"=w231:i32, "Frequency"=w230:dbl)
                  n76 = To Variant(anything=w230) -> (Variant=w229:variant)
                }
                frame "Phase" {
                  n77 = call "From JSON Text.vim"("Data Type and Default Value"=T20 {"Channel"=0, "Phase"=0.0} ("setREF_phi"), "error in (no error)"=w243, "JSON"=w244) -> ("error out"=w242:errorcluster, "Data out"=w241:T20)  [unwired: 7 in]
                  n78 = Unbundle By Name(w241) -> ("Channel"=w240:i32, "Phase"=w239:dbl)
                  n79 = To Variant(anything=w239) -> (Variant=w238:variant)
                }
                frame "TC" {
                  n80 = call "From JSON Text.vim"("Data Type and Default Value"=T21 {"Channel"=0, "TC"=1e-05} ("setREF_phi"), "error in (no error)"=w252, "JSON"=w253) -> ("error out"=w251:errorcluster, "Data out"=w250:T21)  [unwired: 7 in]
                  n81 = Unbundle By Name(w250) -> ("Channel"=w249:i32, "TC"=w248:dbl)
                  n82 = To Variant(anything=w248) -> (Variant=w247:variant)
                }
                frame "RollOff" {
                  n83 = call "From JSON Text.vim"("Data Type and Default Value"=T22 {"Channel"=0, "Roll-Off"=1} ("setREF_Roll-Off"), "error in (no error)"=w261, "JSON"=w262) -> ("error out"=w260:errorcluster, "Data out"=w259:T22)  [unwired: 7 in]
                  n84 = Unbundle By Name(w259) -> ("Channel"=w258:i32, "Roll-Off"=w257:i32)
                  n85 = To Variant(anything=w257) -> (Variant=w256:variant)
                }
              }
              n86 = call "Update REF Parameter.vi"("Parameter"=w220, "error in"=w219, "Value"=w218, "Channel"=w217, "Instrument.Lockin"=w223) -> ("error out"=w221:errorcluster, "Instrument.Lockin out"=w222:refnum<class "Instrument.Lockin.lvclass">)  [unwired: 5 in]
            }
            frame "" {
              n87 = call "From JSON Text.vim"("Data Type and Default Value"=T23 [] ("REF Channels"), "error in (no error)"=w268, "JSON"=w269) -> ("error out"=w264:errorcluster, "Data out"=w265:T23)  [unwired: 7 in]
              n88 = Bundle By Name(cluster=w267, "Cfg_REF"=w265) -> (w266:refnum<class "Instrument.Lockin.lvclass">)
            }
          }
          n89 = Unbundle By Name(w208) -> ("Instrument.DAQ"=w212:refnum<class "Instrument.DAQ.lvclass">, "Cfg_REF"=w206:T23)
          n90 = call "DAQ.setREF.vi"("error in (no error)"=w207, "Channels: Lockin"=w206, "Instrument.DAQ"=w212) -> ("error out"=w210:errorcluster, "Instrument.DAQ out"=w211:refnum<class "Instrument.DAQ.lvclass">)  [unwired: 7 in]
          n91 = call "DAQ.zeroPhase.vi"("error in (no error)"=w210, "Instrument.DAQ"=w211) -> ("error out"=w209:errorcluster)  [unwired: 8 in, 1 out]
        }
        frame "setSweep" {
          n92 = Unbundle By Name(w272) -> ("Sweep"=w271:T50)
          n93 = case shown="\"Time\"" w273 {
            tunnel: w280 -> [w284 w293 w300]
            tunnel: w279 -> [w283 w292 w299]
            tunnel: [w282 w291 w298] -> w278
            tunnel: [w281 w287 w296] -> w270
            tunnel: w271 -> [_ w289 w297]
            frame "", Default {
              w285 = T50 {"Sweep Time (s)"=0.0, "Initial Wait (s)"=0.0, "Return to Start"=FALSE, "Channels"=[]}  # Configure Sweep
              n94 = call "From JSON Text.vim"("Data Type and Default Value"=w285, "error in (no error)"=w283, "JSON"=w284) -> ("error out"=w282:errorcluster, "Data out"=w281:T50)  [unwired: 7 in]
            }
            frame "Time" {
              n95 = call "From JSON Text.vim"("Data Type and Default Value"=T25 {"SweepTime"=0.0} ("setSweep_Time"), "error in (no error)"=w292, "JSON"=w293) -> ("error out"=w291:errorcluster, "Data out"=w288:T25)  [unwired: 7 in]
              n96 = Unbundle By Name(w288) -> ("SweepTime"=w286:dbl)
              n97 = Bundle By Name(cluster=w289, "Sweep Time (s)"=w286) -> (w287:T50)
            }
            frame "Table" {
              n98 = call "From JSON Text.vim"("Data Type and Default Value"=T26[] [] ("Array"), "error in (no error)"=w299, "JSON"=w300) -> ("error out"=w298:errorcluster, "Data out"=w294:T26[])  [unwired: 7 in]
              n99 = call "Replace Sweep Waveforms.vi"("Channels New"=w294, "Sweep in"=w297) -> ("Sweep out"=w296:T50)  [unwired: 9 in]
            }
          }
          n100 = Bundle By Name(cluster=w272, "Sweep"=w270) -> (w276:refnum<class "Instrument.Lockin.lvclass">)
          n101 = Unbundle By Name(w276) -> ("Instrument.DAQ"=w275:refnum<class "Instrument.DAQ.lvclass">, "Sweep"=w274:T50)
          n102 = call "DAQ.setSweep.vi"("error in (no error)"=w278, "setSweep"=w274, "Instrument.DAQ"=w275) -> ("error out"=w277:errorcluster)  [unwired: 7 in, 1 out]
        }
        frame "setSampling" {
          n103 = call "From JSON Text.vim"("Data Type and Default Value"=T27 {"Fs"=204789.0, "#s"=15753}, "error in (no error)"=w308, "JSON"=w310) -> ("error out"=w301:errorcluster, "Data out"=w302:T27)  [unwired: 7 in]
          n104 = Bundle By Name(cluster=w304, "Sampling"=w302) -> (w303:refnum<class "Instrument.Lockin.lvclass">)
          n105 = Unbundle By Name(w303) -> ("Instrument.DAQ"=w307:refnum<class "Instrument.DAQ.lvclass">, "Sampling"=w305:T54)
          n106 = call "DAQ.setSampling.vi"("error in (no error)"=w301, "Sampling"=w305, "Instrument.DAQ"=w307) -> ("error out"=w306:errorcluster)  [unwired: 7 in, 1 out]
        }
        frame "setSamplingFsMode" {
          n107 = call "From JSON Text.vim"("Data Type and Default Value"=T28 {"FsMode"=enum."Manual"} ("setSampleFsMode"), "error in (no error)"=w320, "JSON"=w321) -> ("error out"=w315:errorcluster, "Data out"=w313:T28)  [unwired: 7 in]
          n108 = Unbundle By Name(w313) -> ("FsMode"=w312:T29)
          n109 = Bundle By Name(cluster=w319, "Fs Mode"=w312) -> (w316:refnum<class "Instrument.Lockin.lvclass">)
          n110 = Unbundle By Name(w316) -> ("Instrument.DAQ"=w318:refnum<class "Instrument.DAQ.lvclass">, "Sampling"=w317:T54)
          n111 = call "DAQ.setSampling.vi"("error in (no error)"=w315, "Sampling"=w317, "Instrument.DAQ"=w318) -> ("error out"=w314:errorcluster)  [unwired: 7 in, 1 out]
        }
        frame "setInputGain" {
          n112 = call "From JSON Text.vim"("Data Type and Default Value"=dbl[] [], "error in (no error)"=w333, "JSON"=w334) -> ("error out"=w332:errorcluster, "Data out"=w325:dbl[])  [unwired: 7 in]
          n113 = for {
            tunnel: T30 {"Channel"="AI1", "Gain"=1.0} ("System Cluster") -> [w339]
            tunnel: w325 -> [w338] mode=indexing
            tunnel: [w337] -> w324 mode=indexing
            n114 = Bundle By Name(cluster=w339, "Gain"=w338) -> (w337:T30)
          }
          n115 = Bundle By Name(cluster=w328, "Gain_AI"=w324) -> (w329:refnum<class "Instrument.Lockin.lvclass">)
          n116 = Unbundle By Name(w329) -> ("Instrument.DAQ"=w331:refnum<class "Instrument.DAQ.lvclass">, "Gain_AI"=w323:T48)
          n117 = for {
            tunnel: w323 -> [w336] mode=indexing
            tunnel: [w335] -> w322 mode=indexing
            n118 = Unbundle By Name(w336) -> ("Gain"=w335:dbl)
          }
          n119 = call "DAQ.setInputGain.vi"("error in (no error)"=w332, "Input Gain"=w322, "Instrument.DAQ"=w331) -> ("error out"=w330:errorcluster)  [unwired: 7 in, 1 out]
        }
        frame "setOffset" {
          n120 = call "From JSON Text.vim"("Data Type and Default Value"=dbl[] [], "error in (no error)"=w351, "JSON"=w352) -> ("error out"=w350:errorcluster, "Data out"=w343:dbl[])  [unwired: 7 in]
          n121 = for {
            tunnel: T30 {"Channel"="AI1", "Gain"=1.0} ("System Cluster") -> [w357]
            tunnel: w343 -> [w356] mode=indexing
            tunnel: [w355] -> w342 mode=indexing
            n122 = Bundle By Name(cluster=w357, "Gain"=w356) -> (w355:T30)
          }
          n123 = Bundle By Name(cluster=w346, "Offset_AI"=w342) -> (w347:refnum<class "Instrument.Lockin.lvclass">)
          n124 = Unbundle By Name(w347) -> ("Instrument.DAQ"=w349:refnum<class "Instrument.DAQ.lvclass">, "Offset_AI"=w341:T48)
          n125 = for {
            tunnel: w341 -> [w354] mode=indexing
            tunnel: [w353] -> w340 mode=indexing
            n126 = Unbundle By Name(w354) -> ("Gain"=w353:dbl)
          }
          n127 = call "DAQ.setInputOffset.vi"("error in (no error)"=w350, "Input Offset"=w340, "Instrument.DAQ"=w349) -> ("error out"=w348:errorcluster)  [unwired: 7 in, 1 out]
        }
        frame "setOutputGain" {
          n128 = call "From JSON Text.vim"("Data Type and Default Value"=dbl[] [], "error in (no error)"=w369, "JSON"=w370) -> ("error out"=w364:errorcluster, "Data out"=w361:dbl[])  [unwired: 7 in]
          n129 = for {
            tunnel: T30 {"Channel"="AI1", "Gain"=1.0} ("System Cluster") -> [w375]
            tunnel: w361 -> [w374] mode=indexing
            tunnel: [w373] -> w360 mode=indexing
            n130 = Bundle By Name(cluster=w375, "Gain"=w374) -> (w373:T30)
          }
          n131 = Bundle By Name(cluster=w365, "Gain_AO"=w360) -> (w366:refnum<class "Instrument.Lockin.lvclass">)
          n132 = Unbundle By Name(w366) -> ("Instrument.DAQ"=w368:refnum<class "Instrument.DAQ.lvclass">, "Gain_AO"=w359:T48)
          n133 = for {
            tunnel: w359 -> [w372] mode=indexing
            tunnel: [w371] -> w358 mode=indexing
            n134 = Unbundle By Name(w372) -> ("Gain"=w371:dbl)
          }
          n135 = call "DAQ.setOutputGain.vi"("error in (no error)"=w364, "Output Gain"=w358, "Instrument.DAQ"=w368) -> ("error out"=w367:errorcluster)  [unwired: 7 in, 1 out]
        }
        frame "setDAQ" {
          w390 = -1 items=["Default"=-1, "RSE"=10083, "Differential"=10106, "Pseudodifferential"=12529] ("output terminal configuration")
          w386 = -1 items=["Default"=-1, "RSE"=10083, "NRSE"=10078, "Differential"=10106, "Pseudodifferential"=12529] ("input terminal configuration")
          n136 = call "From JSON Text.vim"("Data Type and Default Value"=T31 [] ("DAQ.Config []"), "error in (no error)"=w392, "JSON"=w393) -> ("error out"=w380:errorcluster, "Data out"=w389:T31)  [unwired: 7 in]
          n137 = call "config UI to not UI (AO and AI).vi"("output terminal configuration"=w390, "input terminal configuration"=w386, "New Ch []"=w389) -> ("AO Config"=w377:T55, "AI Config"=w376:T58)  [unwired: 7 in]
          n138 = Bundle By Name(cluster=w382, "AI"=w376, "AO"=w377) -> (w381:refnum<class "Instrument.Lockin.lvclass">)
          n139 = Unbundle By Name(w381) -> ("Instrument.DAQ"=w383:refnum<class "Instrument.DAQ.lvclass">, "AI"=w385:T58, "Simulation mode"=w378:T39, "AO"=w384:T55)
          n140 = call "DAQ.setAIconfig.vi"("error in (no error)"=w380, "Simulation mode"=w378, "AI Configuration"=w385, "Instrument.DAQ"=w383) -> ("error out"=w388:errorcluster, "Instrument.DAQ out"=w391:refnum<class "Instrument.DAQ.lvclass">)  [unwired: 6 in]
          n141 = call "DAQ.setAOconfig.vi"("error in (no error)"=w388, "AO Configuration"=w384, "Instrument.DAQ"=w391) -> ("error out"=w387:errorcluster)  [unwired: 7 in, 1 out]
        }
        frame "----------LOCAL API----------" {
        }
        frame "showUI" {
          n142 = call "From JSON Text.vim"("Data Type and Default Value"=T36 FALSE ("show UI?"), "error in (no error)"=w400, "JSON"=w403) -> ("error out"=w399:errorcluster, "Data out"=w401:T36)  [unwired: 7 in]
          n143 = Unbundle By Name(w397) -> ("Instrument.DAQ"=w396:refnum<class "Instrument.DAQ.lvclass">)
          n144 = call "DAQ.showUI.vi"("error in (no error)"=w399, "show UI?"=w401, "Instrument.DAQ"=w396) -> ("error out"=w398:errorcluster)  [unwired: 7 in, 1 out]
        }
        frame "setAI" {
          # "Lockin SMO: Set AI"
          n145 = call "From JSON Text.vim"("Data Type and Default Value"=T37 [] ("AI Channels"), "error in (no error)"=w412, "JSON"=w413) -> ("error out"=w406:errorcluster, "Data out"=w404:T37)  [unwired: 7 in]
          n146 = Bundle By Name(cluster=w411, "Cfg_AI"=w404) -> (w405:refnum<class "Instrument.Lockin.lvclass">)
          n147 = Unbundle By Name(w405) -> ("Instrument.DAQ"=w409:refnum<class "Instrument.DAQ.lvclass">, "Cfg_AI"=w408:T37)
          n148 = call "DAQ.setAI.vi"("error in (no error)"=w406, "AI Channels"=w408, "Instrument.DAQ"=w409) -> ("error out"=w407:errorcluster)  [unwired: 7 in, 1 out]
        }
        frame "setData" {
          n149 = case shown="\"DAQ\"" w418 {
            tunnel: w419 -> [w421 w430 w443 w452 w461 w470 w479 w488 w497 w506 w515 w524]
            tunnel: w417 -> [_ w427 w436 w449 w458 w467 w474 w484 w494 w499 w512 w521]
            tunnel: w416 -> [w420 w423 w435 w448 w457 w466 w475 w483 w492 w503 w511 w520]
            tunnel: [w421 w429 w442 w451 w460 w469 w478 w487 w496 w505 w514 w523] -> w415
            tunnel: [w420 w425 w433 w446 w455 w464 w472 w481 w490 w501 w509 w518] -> w414
            frame Default {
            }
            frame "State" {
              n150 = Unbundle By Name(w430) -> ("DAQ State"=w422:T47)
              n151 = Unflatten From String(type=w422, binary string=w427, error in (no error)=w423) -> (value=w428:T47, error out=w426:errorcluster)  [unwired: 2 in, 1 out]
              n152 = Variant To Data(error in=w426, type=w422, Variant=w428) -> (data=w424:T47, error out=w425:errorcluster)
              n153 = Bundle By Name(cluster=w430, "DAQ State"=w424) -> (w429:refnum<class "Instrument.Lockin.lvclass">)
            }
            frame "DAQ" {
              w431 = T31 [] ("DAQ.Config []")
              w441 = -1 items=["Default"=-1, "RSE"=10083, "Differential"=10106, "Pseudodifferential"=12529] ("output terminal configuration")
              w438 = -1 items=["Default"=-1, "RSE"=10083, "NRSE"=10078, "Differential"=10106, "Pseudodifferential"=12529] ("input terminal configuration")
              # "only setData is flatten to string. otherwise use JSON"
              n154 = Unflatten From String(type=w431, binary string=w436, error in (no error)=w435) -> (value=w437:T31, error out=w434:errorcluster)  [unwired: 2 in, 1 out]
              n155 = Variant To Data(error in=w434, type=w431, Variant=w437) -> (data=w432:T31, error out=w433:errorcluster)
              n156 = call "config UI to not UI (AO and AI).vi"("output terminal configuration"=w441, "input terminal configuration"=w438, "New Ch []"=w432) -> ("AO Config"=w440:T55, "AI Config"=w439:T58)  [unwired: 7 in]
              n157 = Bundle By Name(cluster=w443, "AI"=w439, "AO"=w440) -> (w442:refnum<class "Instrument.Lockin.lvclass">)
            }
            frame "Sampling" {
              n158 = Unbundle By Name(w452) -> ("Sampling"=w444:T54)
              n159 = Unflatten From String(type=w444, binary string=w449, error in (no error)=w448) -> (value=w450:T54, error out=w447:errorcluster)  [unwired: 2 in, 1 out]
              n160 = Variant To Data(error in=w447, type=w444, Variant=w450) -> (data=w445:T54, error out=w446:errorcluster)
              n161 = Bundle By Name(cluster=w452, "Sampling"=w445) -> (w451:refnum<class "Instrument.Lockin.lvclass">)
            }
            frame "Waveforms" {
              n162 = Unbundle By Name(w461) -> ("Waveforms"=w453:T60)
              n163 = Unflatten From String(type=w453, binary string=w458, error in (no error)=w457) -> (value=w459:T60, error out=w456:errorcluster)  [unwired: 2 in, 1 out]
              n164 = Variant To Data(error in=w456, type=w453, Variant=w459) -> (data=w454:T60, error out=w455:errorcluster)
              n165 = Bundle By Name(cluster=w461, "Waveforms"=w454) -> (w460:refnum<class "Instrument.Lockin.lvclass">)
            }
            frame "Results" {
              n166 = Unbundle By Name(w470) -> ("Results"=w462:T49)
              n167 = Unflatten From String(type=w462, binary string=w467, error in (no error)=w466) -> (value=w468:T49, error out=w465:errorcluster)  [unwired: 2 in, 1 out]
              n168 = Variant To Data(error in=w465, type=w462, Variant=w468) -> (data=w463:T49, error out=w464:errorcluster)
              n169 = Bundle By Name(cluster=w470, "Results"=w463) -> (w469:refnum<class "Instrument.Lockin.lvclass">)
            }
            frame "SweepWaveforms" {
              n170 = Unbundle By Name(w479) -> ("SweepWaveforms"=w471:T61)
              n171 = Unflatten From String(type=w471, binary string=w474, error in (no error)=w475) -> (value=w477:T61, error out=w473:errorcluster)  [unwired: 2 in, 1 out]
              n172 = Variant To Data(error in=w473, type=w471, Variant=w477) -> (data=w476:T61, error out=w472:errorcluster)
              n173 = Bundle By Name(cluster=w479, "SweepWaveforms"=w476) -> (w478:refnum<class "Instrument.Lockin.lvclass">)
            }
            frame "AOChannels" {
              n174 = Unbundle By Name(w488) -> ("Cfg_AO"=w480:T16)
              n175 = Unflatten From String(type=w480, binary string=w484, error in (no error)=w483) -> (value=w486:T16, error out=w482:errorcluster)  [unwired: 2 in, 1 out]
              n176 = Variant To Data(error in=w482, type=w480, Variant=w486) -> (data=w485:T16, error out=w481:errorcluster)
              n177 = Bundle By Name(cluster=w488, "Cfg_AO"=w485) -> (w487:refnum<class "Instrument.Lockin.lvclass">)
            }
            frame "AIChannels" {
              n178 = Unbundle By Name(w497) -> ("Cfg_AI"=w489:T37)
              n179 = Unflatten From String(type=w489, binary string=w494, error in (no error)=w492) -> (value=w495:T37, error out=w491:errorcluster)  [unwired: 2 in, 1 out]
              n180 = Variant To Data(error in=w491, type=w489, Variant=w495) -> (data=w493:T37, error out=w490:errorcluster)
              n181 = Bundle By Name(cluster=w497, "Cfg_AI"=w493) -> (w496:refnum<class "Instrument.Lockin.lvclass">)
            }
            frame "REFChannels" {
              n182 = Unbundle By Name(w506) -> ("Cfg_REF"=w498:T23)
              n183 = Unflatten From String(type=w498, binary string=w499, error in (no error)=w503) -> (value=w504:T23, error out=w502:errorcluster)  [unwired: 2 in, 1 out]
              n184 = Variant To Data(error in=w502, type=w498, Variant=w504) -> (data=w500:T23, error out=w501:errorcluster)
              n185 = Bundle By Name(cluster=w506, "Cfg_REF"=w500) -> (w505:refnum<class "Instrument.Lockin.lvclass">)
            }
            frame "InputGain" {
              n186 = Unbundle By Name(w515) -> ("Gain_AI"=w507:T48)
              n187 = Unflatten From String(type=w507, binary string=w512, error in (no error)=w511) -> (value=w513:T48, error out=w510:errorcluster)  [unwired: 2 in, 1 out]
              n188 = Variant To Data(error in=w510, type=w507, Variant=w513) -> (data=w508:T48, error out=w509:errorcluster)
              n189 = Bundle By Name(cluster=w515, "Gain_AI"=w508) -> (w514:refnum<class "Instrument.Lockin.lvclass">)
            }
            frame "OutputGain" {
              n190 = Unbundle By Name(w524) -> ("Gain_AO"=w516:T48)
              n191 = Unflatten From String(type=w516, binary string=w521, error in (no error)=w520) -> (value=w522:T48, error out=w519:errorcluster)  [unwired: 2 in, 1 out]
              n192 = Variant To Data(error in=w519, type=w516, Variant=w522) -> (data=w517:T48, error out=w518:errorcluster)
              n193 = Bundle By Name(cluster=w524, "Gain_AO"=w517) -> (w523:refnum<class "Instrument.Lockin.lvclass">)
            }
          }
        }
        frame "autoConfigureDAQ" {
          n194 = Unbundle By Name(w526) -> ("Instrument.DAQ"=w525:refnum<class "Instrument.DAQ.lvclass">)
          n195 = call "DAQ.autoConfigureDAQ.vi"("error in (no error)"=w527, "Instrument.DAQ"=w525) -> ("error out"=w528:errorcluster)  [unwired: 8 in, 1 out]
        }
        frame "setSimulationMode" {
          n196 = call "From JSON Text.vim"("Data Type and Default Value"=Simulation_Mode--enum."AI = noise*AO" ("AI Simulation mode"), "error in (no error)"=w532, "JSON"=w533) -> ("error out"=w531:errorcluster, "Data out"=w529:T39)  [unwired: 7 in]
          n197 = Bundle By Name(cluster=w539, "Simulation mode"=w529) -> (w538:refnum<class "Instrument.Lockin.lvclass">)
          n198 = Unbundle By Name(w538) -> ("Instrument.DAQ"=w537:refnum<class "Instrument.DAQ.lvclass">, "AI"=w536:T58, "Simulation mode"=w535:T39)
          n199 = call "DAQ.setAIconfig.vi"("error in (no error)"=w531, "Simulation mode"=w535, "AI Configuration"=w536, "Instrument.DAQ"=w537) -> ("error out"=w534:errorcluster)  [unwired: 6 in, 1 out]
        }
        frame "setOffsetMode" {
          n200 = Build Array(Offset_Mode--Enum."Remove" ("Offset Mode")) -> (w541:T40[])
          n201 = call "From JSON Text.vim"("Data Type and Default Value"=w541, "error in (no error)"=w543, "JSON"=w546) -> ("error out"=w542:errorcluster, "Data out"=w544:T40[])  [unwired: 7 in]
          n202 = Index Array(array=w544) -> (element=w540:T40)  [unwired: 1 in]
          n203 = Unbundle By Name(w549) -> ("Instrument.DAQ"=w548:refnum<class "Instrument.DAQ.lvclass">)
          n204 = case shown="\"Measure\"" w540 {
            tunnel: w548 -> [w552 w555]
            tunnel: w542 -> [w551 w554]
            tunnel: [w550 w553] -> w547
            frame "Measure" {
              n205 = call "DAQ.measureOffset.vi"("error in (no error)"=w551, "Instrument.DAQ"=w552) -> ("error out"=w550:errorcluster)  [unwired: 8 in, 1 out]
            }
            frame "Remove" {
              n206 = call "DAQ.zeroOffset.vi"("error in (no error)"=w554, "Instrument.DAQ"=w555) -> ("error out"=w553:errorcluster)  [unwired: 8 in, 1 out]
            }
          }
        }
        frame "zeroPhase" {
          n207 = Unbundle By Name(w558) -> ("Instrument.DAQ"=w559:refnum<class "Instrument.DAQ.lvclass">)
          n208 = call "DAQ.zeroPhase.vi"("error in (no error)"=w557, "Instrument.DAQ"=w559) -> ("error out"=w556:errorcluster)  [unwired: 8 in, 1 out]
        }
        frame "setCalibration" {
          n209 = call "From JSON Text.vim"("Data Type and Default Value"=PrivateEvents--DAQ.setCalibration."Check" ("setCalibration"), "error in (no error)"=w560, "JSON"=w564) -> ("error out"=w561:errorcluster, "Data out"=w562:T41)  [unwired: 7 in]
          n210 = Unbundle By Name(w567) -> ("Instrument.DAQ"=w566:refnum<class "Instrument.DAQ.lvclass">)
          n211 = call "DAQ.setCalibration.vi"("error in (no error)"=w561, "setCalibration"=w562, "Instrument.DAQ"=w566) -> ("error out"=w565:errorcluster)  [unwired: 7 in, 1 out]
        }
        frame "setPreFilter" {
          n212 = call "From JSON Text.vim"("Data Type and Default Value"=T42 {"60 Hz"=FALSE, "Low Pass"=FALSE, "Low Pass Cutoff (Hz)"=0.0} ("PreFilter"), "error in (no error)"=w569, "JSON"=w571) -> ("error out"=w568:errorcluster, "Data out"=w570:T42)  [unwired: 7 in]
          n213 = Bundle By Name(cluster=w574, "Prefilter"=w570) -> (w575:refnum<class "Instrument.Lockin.lvclass">)
          n214 = Unbundle By Name(w575) -> ("Instrument.DAQ"=w577:refnum<class "Instrument.DAQ.lvclass">, "Prefilter"=w573:T42)
          n215 = call "DAQ.setPreFilter.vi"("error in (no error)"=w568, "PreFilter"=w573, "Instrument.DAQ"=w577) -> ("error out"=w576:errorcluster)  [unwired: 7 in, 1 out]
        }
        frame "setLinkFrequencies" {
          n216 = call "From JSON Text.vim"("Data Type and Default Value"=T43 {"Link?"=FALSE, "Frequency (Hz)"=0.0} ("Link Frequencies"), "error in (no error)"=w580, "JSON"=w582) -> ("error out"=w579:errorcluster, "Data out"=w578:T43)  [unwired: 7 in]
          n217 = Bundle By Name(cluster=w586, "Link Frequencies"=w578) -> (w587:refnum<class "Instrument.Lockin.lvclass">)
          n218 = Unbundle By Name(w587) -> ("Instrument.DAQ"=w585:refnum<class "Instrument.DAQ.lvclass">, "Link Frequencies"=w584:T43)
          n219 = call "DAQ.setLinkFrequencies.vi"("error in (no error)"=w579, "Link Frequencies"=w584, "Instrument.DAQ"=w585) -> ("error out"=w583:errorcluster)  [unwired: 7 in, 1 out]
        }
        frame "setLimitAmplitude" {
          w591 = T62 {"Limit?"=FALSE, "Limit (V)"=0.0}  # Limit Amplitude
          n220 = call "From JSON Text.vim"("Data Type and Default Value"=w591, "error in (no error)"=w589, "JSON"=w592) -> ("error out"=w588:errorcluster, "Data out"=w590:T62)  [unwired: 7 in]
          n221 = Bundle By Name(cluster=w596, "Amplitude Limit"=w590) -> (w597:refnum<class "Instrument.Lockin.lvclass">)
          n222 = Unbundle By Name(w597) -> ("Instrument.DAQ"=w595:refnum<class "Instrument.DAQ.lvclass">, "Amplitude Limit"=w594:T62)
          n223 = call "DAQ.setAmplitudeLimit.vi"("error in (no error)"=w588, "Amplitude Limit"=w594, "Instrument.DAQ"=w595) -> ("error out"=w593:errorcluster)  [unwired: 7 in, 1 out]
        }
        frame "setSamplingDecimationPreDSP" {
          n224 = call "From JSON Text.vim"("Data Type and Default Value"=0, "error in (no error)"=w601, "JSON"=w602) -> ("error out"=w600:errorcluster, "Data out"=w599:i32)  [unwired: 7 in]
          n225 = Bundle By Name(cluster=w604, "Decimation.PreDSP"=w599) -> (w603:refnum<class "Instrument.Lockin.lvclass">)
          n226 = Unbundle By Name(w603) -> ("Instrument.DAQ"=w607:refnum<class "Instrument.DAQ.lvclass">, "Sampling"=w606:T54)
          n227 = call "DAQ.setSampling.vi"("error in (no error)"=w600, "Sampling"=w606, "Instrument.DAQ"=w607) -> ("error out"=w605:errorcluster)  [unwired: 7 in, 1 out]
        }
        frame "setSamplingDecimationPostDSP" {
          n228 = call "From JSON Text.vim"("Data Type and Default Value"=0, "error in (no error)"=w611, "JSON"=w612) -> ("error out"=w610:errorcluster, "Data out"=w609:i32)  [unwired: 7 in]
          n229 = Bundle By Name(cluster=w614, "Decimation.PreDSP"=w609) -> (w613:refnum<class "Instrument.Lockin.lvclass">)
          n230 = Unbundle By Name(w613) -> ("Instrument.DAQ"=w617:refnum<class "Instrument.DAQ.lvclass">, "Sampling"=w616:T54)
          n231 = call "DAQ.setSampling.vi"("error in (no error)"=w610, "Sampling"=w616, "Instrument.DAQ"=w617) -> ("error out"=w615:errorcluster)  [unwired: 7 in, 1 out]
        }
        frame "setSamplingMode" {
          (unwired) DAQ.Sampling.Fs_Mode--enum."Manual"  # Fs Mode
          # "#todo\nAUTO sampling mode"
          n232 = call "From JSON Text.vim"("Data Type and Default Value"=T44 {"SampleMode"=10123} ("setSampleMode"), "error in (no error)"=w622, "JSON"=w623) -> ("error out"=w621:errorcluster, "Data out"=w619:T44)  [unwired: 7 in]
          n233 = Unbundle By Name(w619) -> ("SampleMode"=w618:T45)
          n234 = Bundle By Name(cluster=w628, "sample mode"=w618) -> (w625:refnum<class "Instrument.Lockin.lvclass">)
          n235 = Unbundle By Name(w625) -> ("Instrument.DAQ"=w627:refnum<class "Instrument.DAQ.lvclass">, "Sampling"=w626:T54)
          n236 = call "DAQ.setSampling.vi"("error in (no error)"=w621, "Sampling"=w626, "Instrument.DAQ"=w627) -> ("error out"=w624:errorcluster)  [unwired: 7 in, 1 out]
        }
        frame "setSamplingFsMultiplier" {
          n237 = call "From JSON Text.vim"("Data Type and Default Value"=0.0, "error in (no error)"=w630, "JSON"=w632) -> ("error out"=w629:errorcluster, "Data out"=w631:dbl)  [unwired: 7 in]
          n238 = Bundle By Name(cluster=w638, "Fs Multiplier"=w631) -> (w635:refnum<class "Instrument.Lockin.lvclass">)
          n239 = Unbundle By Name(w635) -> ("Instrument.DAQ"=w637:refnum<class "Instrument.DAQ.lvclass">, "Sampling"=w636:T54)
          n240 = call "DAQ.setSampling.vi"("error in (no error)"=w629, "Sampling"=w636, "Instrument.DAQ"=w637) -> ("error out"=w634:errorcluster)  [unwired: 7 in, 1 out]
        }
        frame "setSamplingFsOutput" {
          n241 = call "From JSON Text.vim"("Data Type and Default Value"=0.0, "error in (no error)"=w641, "JSON"=w642) -> ("error out"=w640:errorcluster, "Data out"=w639:dbl)  [unwired: 7 in]
          n242 = Bundle By Name(cluster=w648, "Fs.Output"=w639) -> (w645:refnum<class "Instrument.Lockin.lvclass">)
          n243 = Unbundle By Name(w645) -> ("Instrument.DAQ"=w647:refnum<class "Instrument.DAQ.lvclass">, "Sampling"=w646:T54)
          n244 = call "DAQ.setSampling.vi"("error in (no error)"=w640, "Sampling"=w646, "Instrument.DAQ"=w647) -> ("error out"=w644:errorcluster)  [unwired: 7 in, 1 out]
        }
        frame "setSamplingRefreshRate" {
          n245 = call "From JSON Text.vim"("Data Type and Default Value"=0.0, "error in (no error)"=w650, "JSON"=w653) -> ("error out"=w649:errorcluster, "Data out"=w651:dbl)  [unwired: 7 in]
          n246 = Bundle By Name(cluster=w658, "Refresh Rate (Hz)"=w651) -> (w655:refnum<class "Instrument.Lockin.lvclass">)
          n247 = Unbundle By Name(w655) -> ("Instrument.DAQ"=w657:refnum<class "Instrument.DAQ.lvclass">, "Sampling"=w656:T54)
          n248 = call "DAQ.setSampling.vi"("error in (no error)"=w649, "Sampling"=w656, "Instrument.DAQ"=w657) -> ("error out"=w654:errorcluster)  [unwired: 7 in, 1 out]
        }
      }
    }
    frame Error {
    }
  }
  "error out" <- w7
  "Instrument.Lockin out" <- w6
  "Command" <- w3
  "Processed Data" <- w5
